vi "Name Folder Path.vi"(10 "Name":string) -> (2 "Name Folder Path":path)   [LabVIEW 2021, in "_Rename.lvlib" / "Script.lvlib" / "Script.lvclass"]
uses:
  Script/Script/Script.lvclass
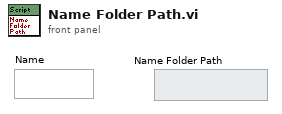
[diagram p1: front panel]
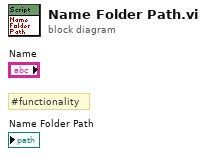
[diagram p0: block diagram]
diagram:
  # "#functionality"
